vi "UpdateRefreshTimes.vi"(8 "error in (no error)":errorcluster, 10 "Update Time":bool=TRUE, 11 "ControlState in":T1 {"ChainMask" format="0x%02x"}) -> (0 "error out":errorcluster, 3 "ControlState out":T1 {"ChainMask" format="0x%02x"})   [LabVIEW 2025, in "ArduinoSerialBling.lvlib"]
uses:
  ArduinoSerialBling.lvlib
  ControlState.ctl
  ConnectionType.ctl
  UdpConnection.ctl
  ChainState.ctl
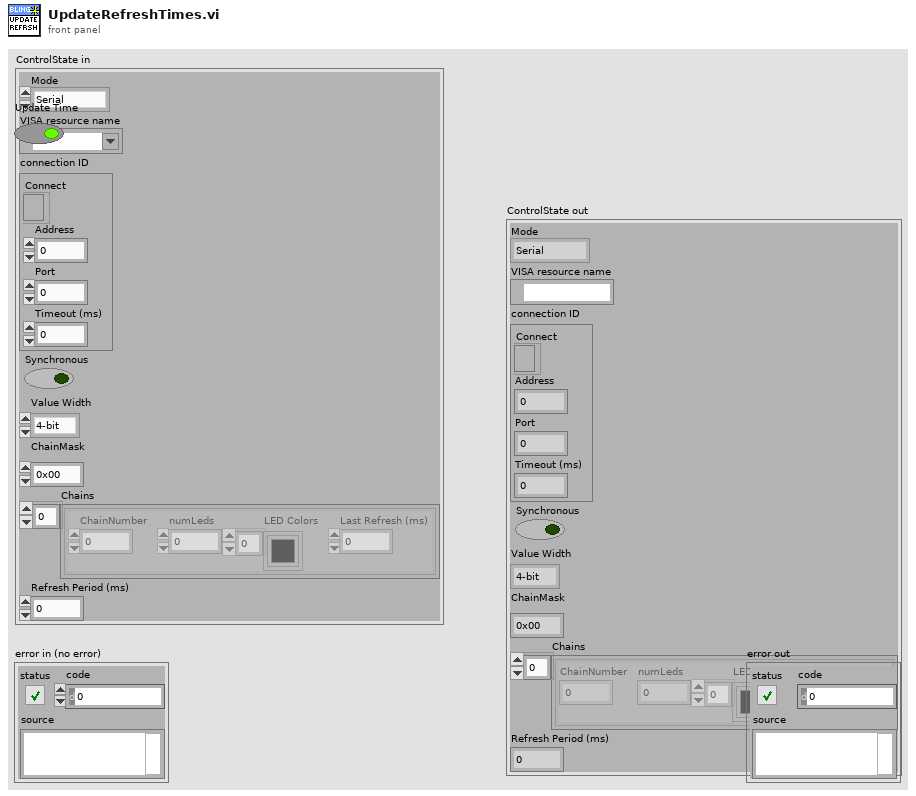
[diagram p1: front panel]
types:
  T1 = typedef "ArduinoSerialBling.lvlib/ControlState.ctl" = cluster{"Mode":T2, "VISA resource name":refnum<visa-resource-name>, "connection ID":T3, "Synchronous":bool, "Value Width":enum16{"4-bit", "8-bit"}, "ChainMask":u8, "Chains":T4[], "Refresh Period (ms)":u32}
  T2 = typedef "ConnectionType.ctl" = enum16{"Serial", "Ethernet", "Offline"}
  T3 = typedef "UdpConnection.ctl" = cluster{"Connect":refnum<k16>, "Address":u32, "Port":u16, "Timeout (ms)":i32}
  T4 = typedef "ArduinoSerialBling.lvlib/ChainState.ctl" = cluster{"ChainNumber":u8, "numLeds":u8, "LED Colors":u32[], "Last Refresh (ms)":u32}
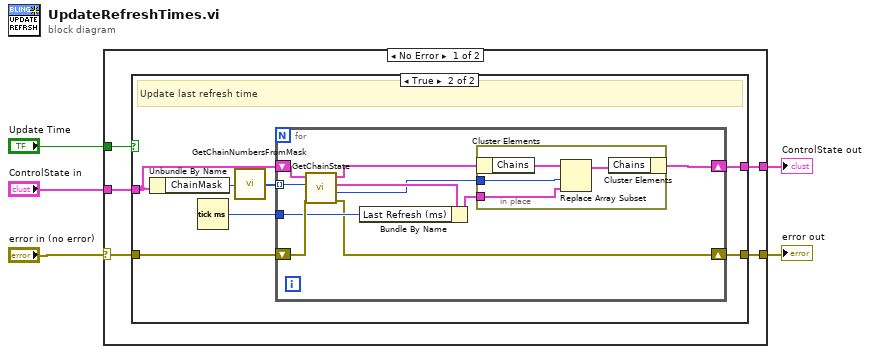
[diagram p0: block diagram]
diagram:
  n1 = case shown="No Error" "error in (no error)" {
    selector: "error in (no error)" -> [w9 w34]
    tunnel: [w7 w35] -> w4
    tunnel: "ControlState in" -> [w6 w35]
    tunnel: [w8 w34] -> w2
    tunnel: "Update Time" -> [w10 _]
    frame No Error {
      n2 = case shown="True" w10 {
        tunnel: w9 -> [w12 w16]
        tunnel: [w12 w13] -> w8
        tunnel: [w11 w14] -> w7
        tunnel: w6 -> [w11 w17]
        frame False {
        }
        frame True {
          # "Update last refresh time"
          n3 = Unbundle By Name(w17) -> ("ChainMask"=w19:u8)
          n4 = Tick Count (ms)() -> (millisecond timer value=w15:u32)
          n5 = call "GetChainNumbersFromMask.vi"("ChainMask"=w19) -> ("Chains"=w18:u8[])
          n6 = for {
            tunnel: w18 -> [w28] mode=indexing
            tunnel: w15 -> [w26]
            shift-right: [w21] -> w14
            shift-left: w17 -> [w25]
            shift-right: [w22] -> w13
            shift-left: w16 -> [w29]
            n7 = call "GetChainState.vi"("error in (no error)"=w29, "ChainNumber"=w28, "ControlState in"=w25) -> ("error out"=w22:errorcluster, "ChainIndex"=w24:i32, "ChainState"=w27:T4, "ControlState out"=w20:T1)  [unwired: 5 in]
            n8 = Bundle By Name(cluster=w27, "Last Refresh (ms)"=w26) -> (w23:T4)
            n9 = in-place {
              in-place-border: w24 -> [w31]
              in-place-border: w23 -> [w30]
              n10 = in-place-cluster #1(w20) -> ("Chains"=w33:T4[])
              n11 = Replace Array Subset(array=w33, new element=w30, index=w31) -> (w32:T4[])
              n12 = in-place-cluster #1("Chains"=w32) -> (w21:T1)
            }
          }
        }
      }
    }
    frame Error {
    }
  }
  "ControlState out" <- w4
  "error out" <- w2
